vi "Configure Trigger Setup.vi"(4 "HF Reject (OFF)":bool, 6 "Trigger Coupling (0 : DC)":u16(ring) items=["DC", "AC", "LF Reject", "HF Reject"], 7 "Trigger Type (0: Edge)":u16(ring) items=["Edge", "Pulse", "Video", "Pattern", "Duration"], 8 "error in (no error)":errorcluster, 9 "Trigger Holdoff (500E-9)":dbl=5e-07 format="%^#_6g", 10 "Trigger Sensitivity (0.3div)":dbl=0.3 format="%^#_6g", 11 "VISA resource name":refnum<visa-resource-name>) -> (0 "error out":errorcluster, 3 "VISA resource name out":refnum<visa-resource-name>)   [LabVIEW 2015, in "RIGOL DS1000 Series.lvlib"]
doc: "Configures trigger setup of the oscilloscope.\n\n<b>Note:</b>\n\nThis VI only applies to the Rigol DS1000B and DS1000D Series models."
uses:
  RIGOL DS1000 Series.lvlib
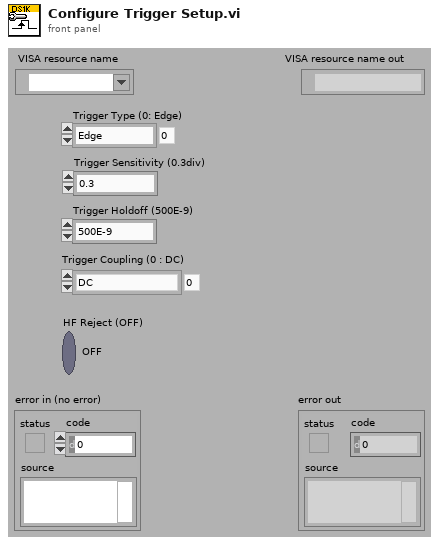
[diagram p1: front panel]
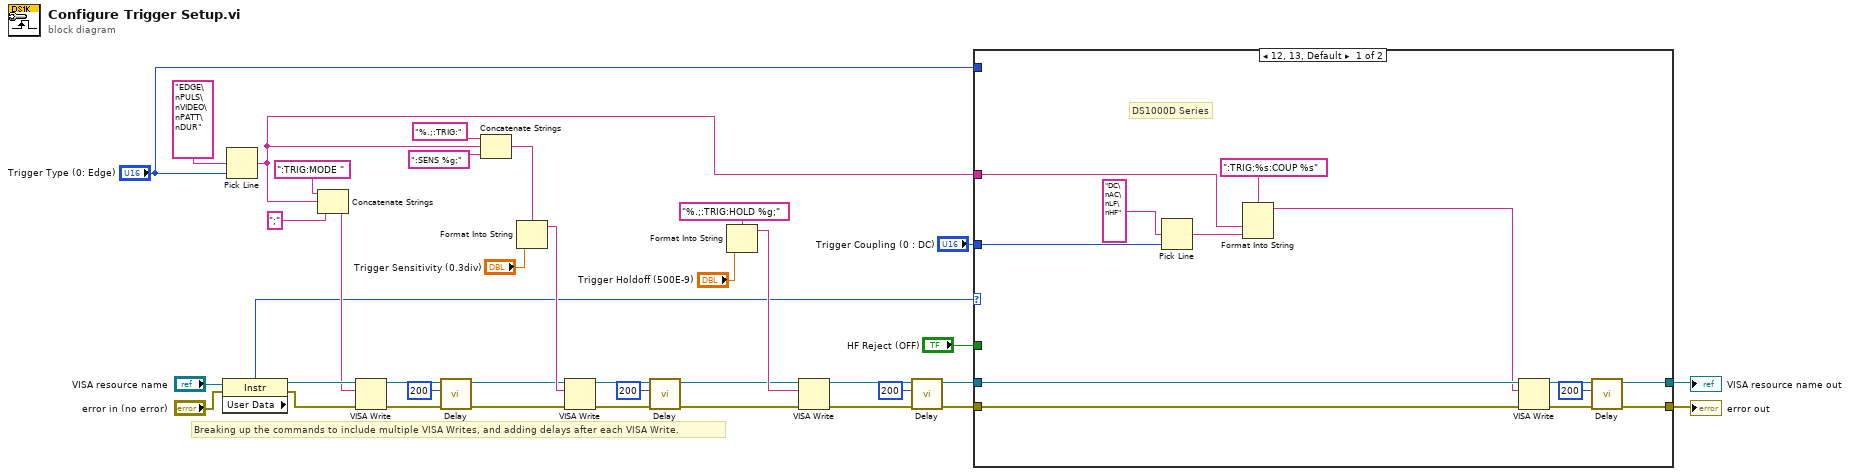
[diagram p0: block diagram]
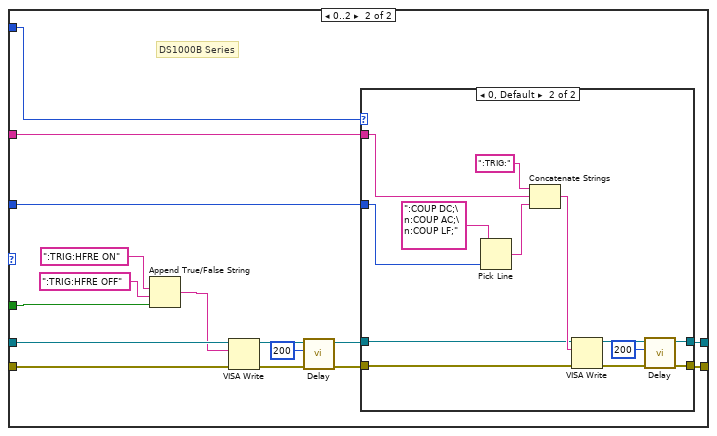
[diagram p2: hidden frame]
diagram:
  # "Breaking up the commands to include multiple VISA Writes, and adding delays after each VISA Write."
  n1 = property class="Instr"(reference="VISA resource name", error in="error in (no error)") -> (reference out=w23:refnum<visa-resource-name>, error out=w22:errorcluster, "User Data"=w2:u32)
  n2 = Pick Line(multi-line string="EDGE\nPULS\nVIDEO\nPATT\nDUR", line index="Trigger Type (0: Edge)") -> (output string=w27:string)  [unwired: 1 out]
  n3 = Concatenate Strings(":TRIG:MODE " ("string (\"\")"), w27, ";" ("string")) -> (w21:string)
  n4 = VISA Write(VISA resource name=w23, write buffer=w21, error in (no error)=w22) -> (VISA resource name out=w20:refnum<visa-resource-name>, error out=w19:errorcluster)  [unwired: 1 out]
  n5 = call "Delay.vi"("error in (no error)"=w19, "Delay (ms)"=u32 200, "VISA resource name"=w20) -> ("error out"=w14:errorcluster, "VISA resource name out"=w15:refnum<visa-resource-name>)  [unwired: 7 out]
  n6 = Concatenate Strings("%.;:TRIG:" ("string"), w27, ":SENS %g;" ("string")) -> (w29:string)
  n7 = Format Into String(format string=w29, "Trigger Sensitivity (0.3div)") -> (resulting string=w16:string)  [unwired: 2 in, 1 out]
  n8 = VISA Write(VISA resource name=w15, write buffer=w16, error in (no error)=w14) -> (VISA resource name out=w18:refnum<visa-resource-name>, error out=w17:errorcluster)  [unwired: 1 out]
  n9 = call "Delay.vi"("error in (no error)"=w17, "Delay (ms)"=u32 200, "VISA resource name"=w18) -> ("error out"=w11:errorcluster, "VISA resource name out"=w12:refnum<visa-resource-name>)  [unwired: 7 out]
  n10 = Format Into String(format string="%.;:TRIG:HOLD %g;" ("Level Command"), "Trigger Holdoff (500E-9)") -> (resulting string=w13:string)  [unwired: 2 in, 1 out]
  n11 = VISA Write(VISA resource name=w12, write buffer=w13, error in (no error)=w11) -> (VISA resource name out=w10:refnum<visa-resource-name>, error out=w9:errorcluster)  [unwired: 1 out]
  n12 = call "Delay.vi"("error in (no error)"=w9, "Delay (ms)"=u32 200, "VISA resource name"=w10) -> ("error out"=w3:errorcluster, "VISA resource name out"=w4:refnum<visa-resource-name>)  [unwired: 7 out]
  n13 = case shown="12, 13, Default" w2 {
    tunnel: "Trigger Coupling (0 : DC)" -> [w50 w67]
    tunnel: "Trigger Type (0: Edge)" -> [_ w66]
    tunnel: w27 -> [w48 w65]
    tunnel: "HF Reject (OFF)" -> [_ w64]
    tunnel: [w40 w62] -> w8
    tunnel: w4 -> [w43 w58]
    tunnel: w3 -> [w42 w57]
    tunnel: [w41 w63] -> w1
    frame 12, 13, Default {
      # "DS1000D Series"
      n14 = Pick Line(multi-line string="DC\nAC\nLF\nHF", line index=w50) -> (output string=w49:string)  [unwired: 1 out]
      n15 = Format Into String(format string=":TRIG:%s:COUP %s", w48, w49) -> (resulting string=w39:string)  [unwired: 2 in, 1 out]
      n16 = VISA Write(VISA resource name=w43, write buffer=w39, error in (no error)=w42) -> (VISA resource name out=w45:refnum<visa-resource-name>, error out=w44:errorcluster)  [unwired: 1 out]
      n17 = call "Delay.vi"("error in (no error)"=w44, "Delay (ms)"=u32 200, "VISA resource name"=w45) -> ("error out"=w40:errorcluster, "VISA resource name out"=w41:refnum<visa-resource-name>)  [unwired: 7 out]
    }
    frame 0..2 {
      # "DS1000B Series"
      n18 = Append True/False String(1:w64, 2:":TRIG:HFRE OFF" ("false string"), 3:":TRIG:HFRE ON" ("true string")) -> (0:w56:string)  [unwired: 1 out]
      n19 = VISA Write(VISA resource name=w58, write buffer=w56, error in (no error)=w57) -> (VISA resource name out=w60:refnum<visa-resource-name>, error out=w59:errorcluster)  [unwired: 1 out]
      n20 = call "Delay.vi"("error in (no error)"=w59, "Delay (ms)"=u32 200, "VISA resource name"=w60) -> ("error out"=w54:errorcluster, "VISA resource name out"=w55:refnum<visa-resource-name>)  [unwired: 7 out]
      n21 = case shown="0, Default" w66 {
        tunnel: w67 -> [_ w81]
        tunnel: w65 -> [_ w79]
        tunnel: w55 -> [w69 w71]
        tunnel: w54 -> [w68 w70]
        tunnel: [w69 w74] -> w63
        tunnel: [w68 w73] -> w62
        frame 2 {
        }
        frame 0, Default {
          n22 = Pick Line(multi-line string=":COUP DC;\n:COUP AC;\n:COUP LF;", line index=w81) -> (output string=w78:string)  [unwired: 1 out]
          n23 = Concatenate Strings(":TRIG:" ("string"), w79, w78) -> (w75:string)
          n24 = VISA Write(VISA resource name=w71, write buffer=w75, error in (no error)=w70) -> (VISA resource name out=w76:refnum<visa-resource-name>, error out=w77:errorcluster)  [unwired: 1 out]
          n25 = call "Delay.vi"("error in (no error)"=w77, "Delay (ms)"=u32 200, "VISA resource name"=w76) -> ("error out"=w73:errorcluster, "VISA resource name out"=w74:refnum<visa-resource-name>)  [unwired: 7 out]
        }
      }
    }
  }
  "error out" <- w8
  "VISA resource name out" <- w1
